vi "Get Internal Command Data References.vi"(8 "error in (no error)":errorcluster, 11 "Item Ref in":T1 format="%.0x") -> (0 "error out":errorcluster, 1 "Refs":T2(array[cluster]) {"VS Refs" format="%.0x"}, 2 "Internal Command Engine References":T3, 3 "Item Ref out":T1 format="%.0x")   [LabVIEW 2015, in "J1939 Addon System Explorer.lvlib"]
uses:
  J1939 Addon System Explorer.lvlib
  <vilib>/NI Veristand/Custom Device API/Custom Device Item Ref.ctl
  Shared/Types/SysDef Command Settings.ctl
  <vilib>/NI Veristand/Custom Device Tools/Custom Device Utility Library/NI VeriStand - Search for Item by Name.vi
  Shared/SubVIs/Constants.vi
  <vilib>/NI Veristand/Custom Device Tools/Custom Device Utility Library/Custom Device Utility Library.lvlib
  Shared/J1939 Addon Shared.lvlib
  <vilib>/NI VeriStand/Custom Device API/Custom Device API.lvlib
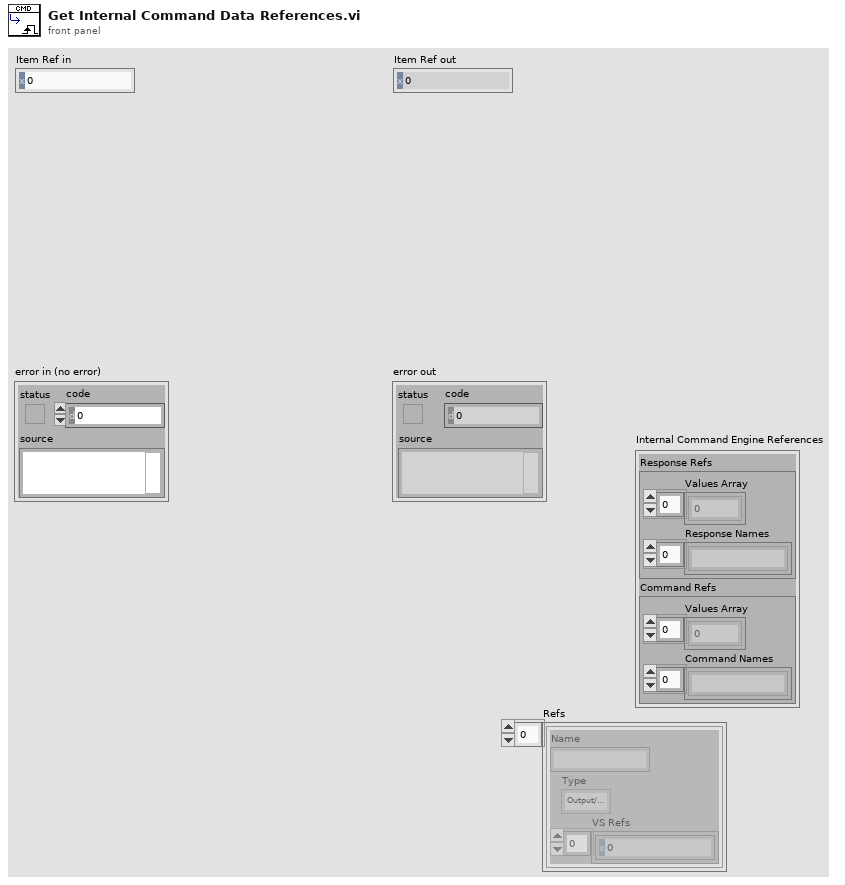
[diagram p1: front panel]
types:
  T1 = typedef "Custom Device API.lvlib/Custom Device Item Ref.ctl" = u64
  T2 = cluster{"Name":string, "Type":enum16{"Output/Write", "Input/Read", "Input/ReadWrite"}, "VS Refs":T1[]}[]
  T3 = typedef "J1939 Addon Shared.lvlib/SysDef Command Settings.ctl" = cluster{"Response Refs":cluster{"Values Array":dbl[], "Response Names":string[]}, "Command Refs":cluster{"Values Array":dbl[], "Command Names":string[]}}
  T4 = enum16{"Output/Write", "Input/Read", "Input/ReadWrite"}
  T5 = cluster{"Name":string, "Type":enum16{"Output/Write", "Input/Read", "Input/ReadWrite"}, "VS Refs":T1[]}
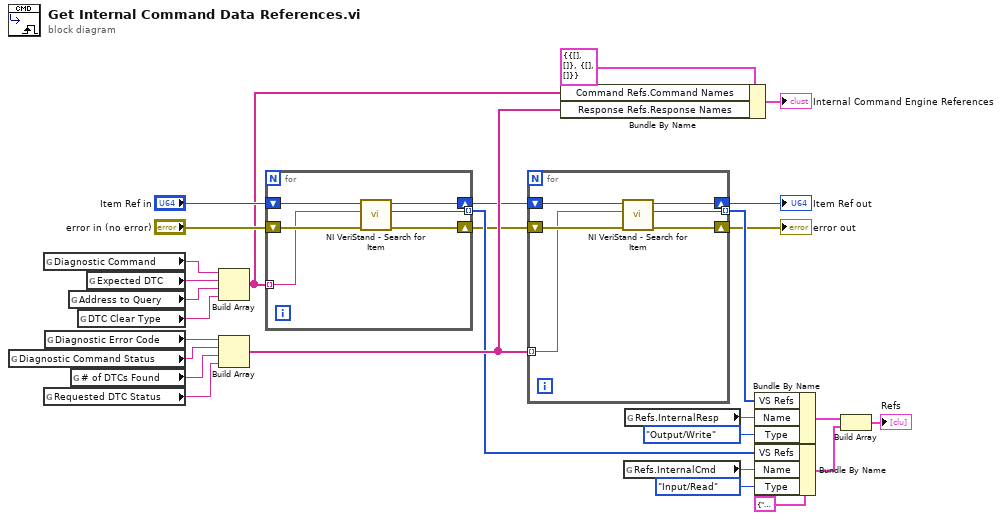
[diagram p0: block diagram]
diagram:
  w4 = T5 {"Name"="", "Type"=enum."Output/Write", "VS Refs"=[]} ("Group")
  n1 = global read "Constants.vi" "Diagnostic Command Status"() -> (w21:string)
  n2 = global read "Constants.vi" "Diagnostic Command"() -> (w28:string)
  n3 = global read "Constants.vi" "Requested DTC Status"() -> (w23:string)
  n4 = global read "Constants.vi" "Diagnostic Error Code"() -> (w20:string)
  n5 = global read "Constants.vi" "Address to Query"() -> (w26:string)
  n6 = global read "Constants.vi" "# of DTCs Found"() -> (w22:string)
  n7 = global read "Constants.vi" "DTC Clear Type"() -> (w25:string)
  n8 = global read "Constants.vi" "Expected DTC"() -> (w27:string)
  n9 = Build Array(w28, w27, w26, w25) -> (w17:string[])
  n10 = Build Array(w20, w21, w22, w23) -> (w16:string[])
  n11 = for {
    tunnel: [w34] -> w7 mode=indexing
    tunnel: w17 -> [w29] mode=indexing
    shift-right: [w32] -> w6
    shift-left: "error in (no error)" -> [w33]
    shift-right: [w31] -> w5
    shift-left: "Item Ref in" -> [w30]
    n12 = call-poly <vilib>:"NI VeriStand - Search for Item.vi"("error in"=w33, "Item Name"=w29, "Section Ref in"=w30) -> ("error out"=w32:errorcluster, "Item Ref"=w34:T1, "Section Ref out"=w31:T1)  [unwired: 5 in, 1 out]
  }
  n13 = for {
    tunnel: [w39] -> w12 mode=indexing
    tunnel: w16 -> [w35] mode=indexing
    shift-right: [w37] -> w10
    shift-left: w6 -> [w38]
    shift-right: [w36] -> w11
    shift-left: w5 -> [w40]
    n14 = call-poly <vilib>:"NI VeriStand - Search for Item.vi"("error in"=w38, "Item Name"=w35, "Section Ref in"=w40) -> ("error out"=w37:errorcluster, "Item Ref"=w39:T1, "Section Ref out"=w36:T1)  [unwired: 5 in, 1 out]
  }
  "Item Ref out" <- w11
  "error out" <- w10
  n15 = Bundle By Name(cluster=T3 {"Response Refs"={"Values Array"=[], "Response Names"=[]}, "Command Refs"={"Values Array"=[], "Command Names"=[]}} ("Internal Command Engine References"), "Command Refs.Command Names"=w17, "Response Refs.Response Names"=w16) -> (→"Internal Command Engine References":T3)
  n16 = global read "Constants.vi" "Refs.InternalCmd"() -> (w8:string)
  n17 = global read "Constants.vi" "Refs.InternalResp"() -> (w14:string)
  n18 = Bundle By Name(cluster=w4, "VS Refs"=w12, "Name"=w14, "Type"=T4."Output/Write") -> (w3:T5)
  n19 = Bundle By Name(cluster=w4, "VS Refs"=w7, "Name"=w8, "Type"=T4."Input/Read") -> (w2:T5)
  n20 = Build Array(w3, w2) -> (→"Refs":T2)
